vi "Control Panel.vi"(8 "error in (no error)":errorcluster, 11 "LCD Retarder in":refnum<class "LCD Retarder.lvclass">) -> (0 "error out":errorcluster, 3 "LCD Retarder out":refnum<class "LCD Retarder.lvclass">)   [LabVIEW 2017, in "LCD Retarder.lvclass"]
uses:
  LCD Retarder.lvclass
  LCD Retarder.lvclass/LCD Retarder.ctl
  <vilib>/DAQmx/write.llb/DAQmx Write (Analog DBL 1Chan 1Samp).vi
  <vilib>/DAQmx/create/channels.llb/DAQmx Create Channel (AO-Voltage-Basic).vi
  <vilib>/DAQmx/miscellaneous.llb/DAQmx Fill In Error Info.vi
  Main/Global/Flags.vi
  Utility Classes/Readable/Readable.lvclass
panel:
  in  "Analog \nOutput \nSync":bool
  in  "Alternate":bool
  in  "Frequency":dbl=0.01 min=0.01 max=6.0
  out "?":bool
  out "?":bool
  in  "Retardance 2":dbl
  in  "Retardance 1":dbl
  in  "stop":bool
  out "error":bool caption="Error"
  in  "Check for Instrument":bool
  out "Current Retardance":dbl[unit] caption="Retardance"
  out "Ready":bool
  in  "waveoptions":T1(radio) caption="Wave Options"
  in  "Wavelength":dbl[unit]=7.81e-07
  out "Title":string="LCD Retarder Control Program"
  in  "Zero":bool
  in  "Set\nRetardance":bool
  in  "Goto Retardance":dbl[unit]
  in  "Exit":bool
  # "and"
  # "at"
  # "Hz"
  # "between"
  # "Note from John: Analog Output #0 will toggle from 0 to 1 V in synch with this."
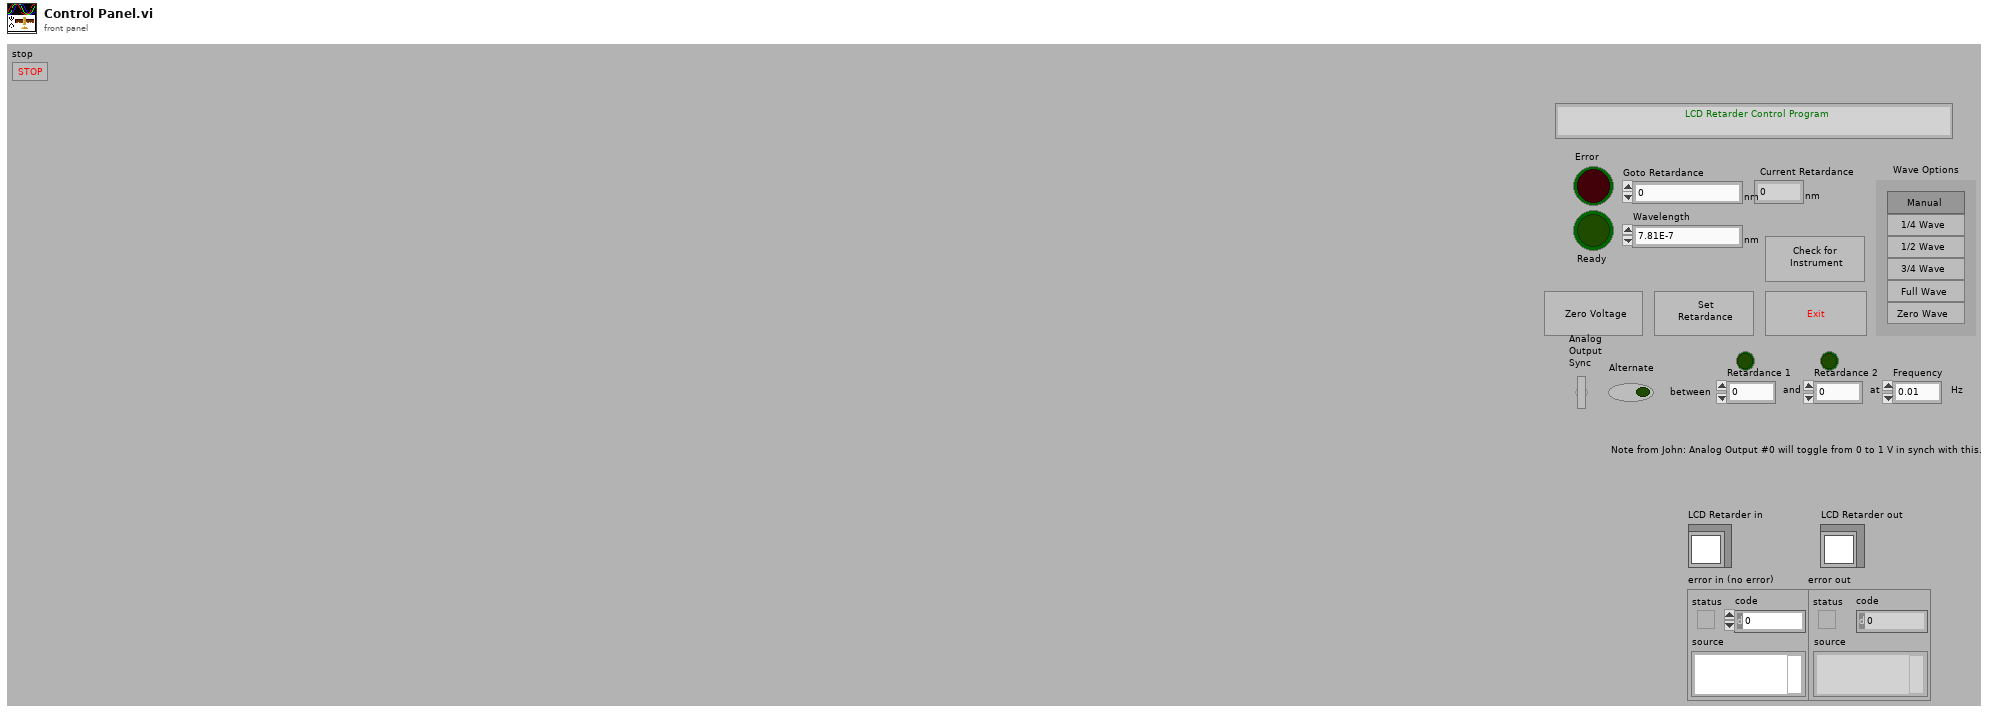
[diagram p1: front panel]
types:
  T1 = enum32{"Manual", "1/4 Wave", "1/2 Wave", "3/4 Wave", "Full Wave", "Zero Wave"}
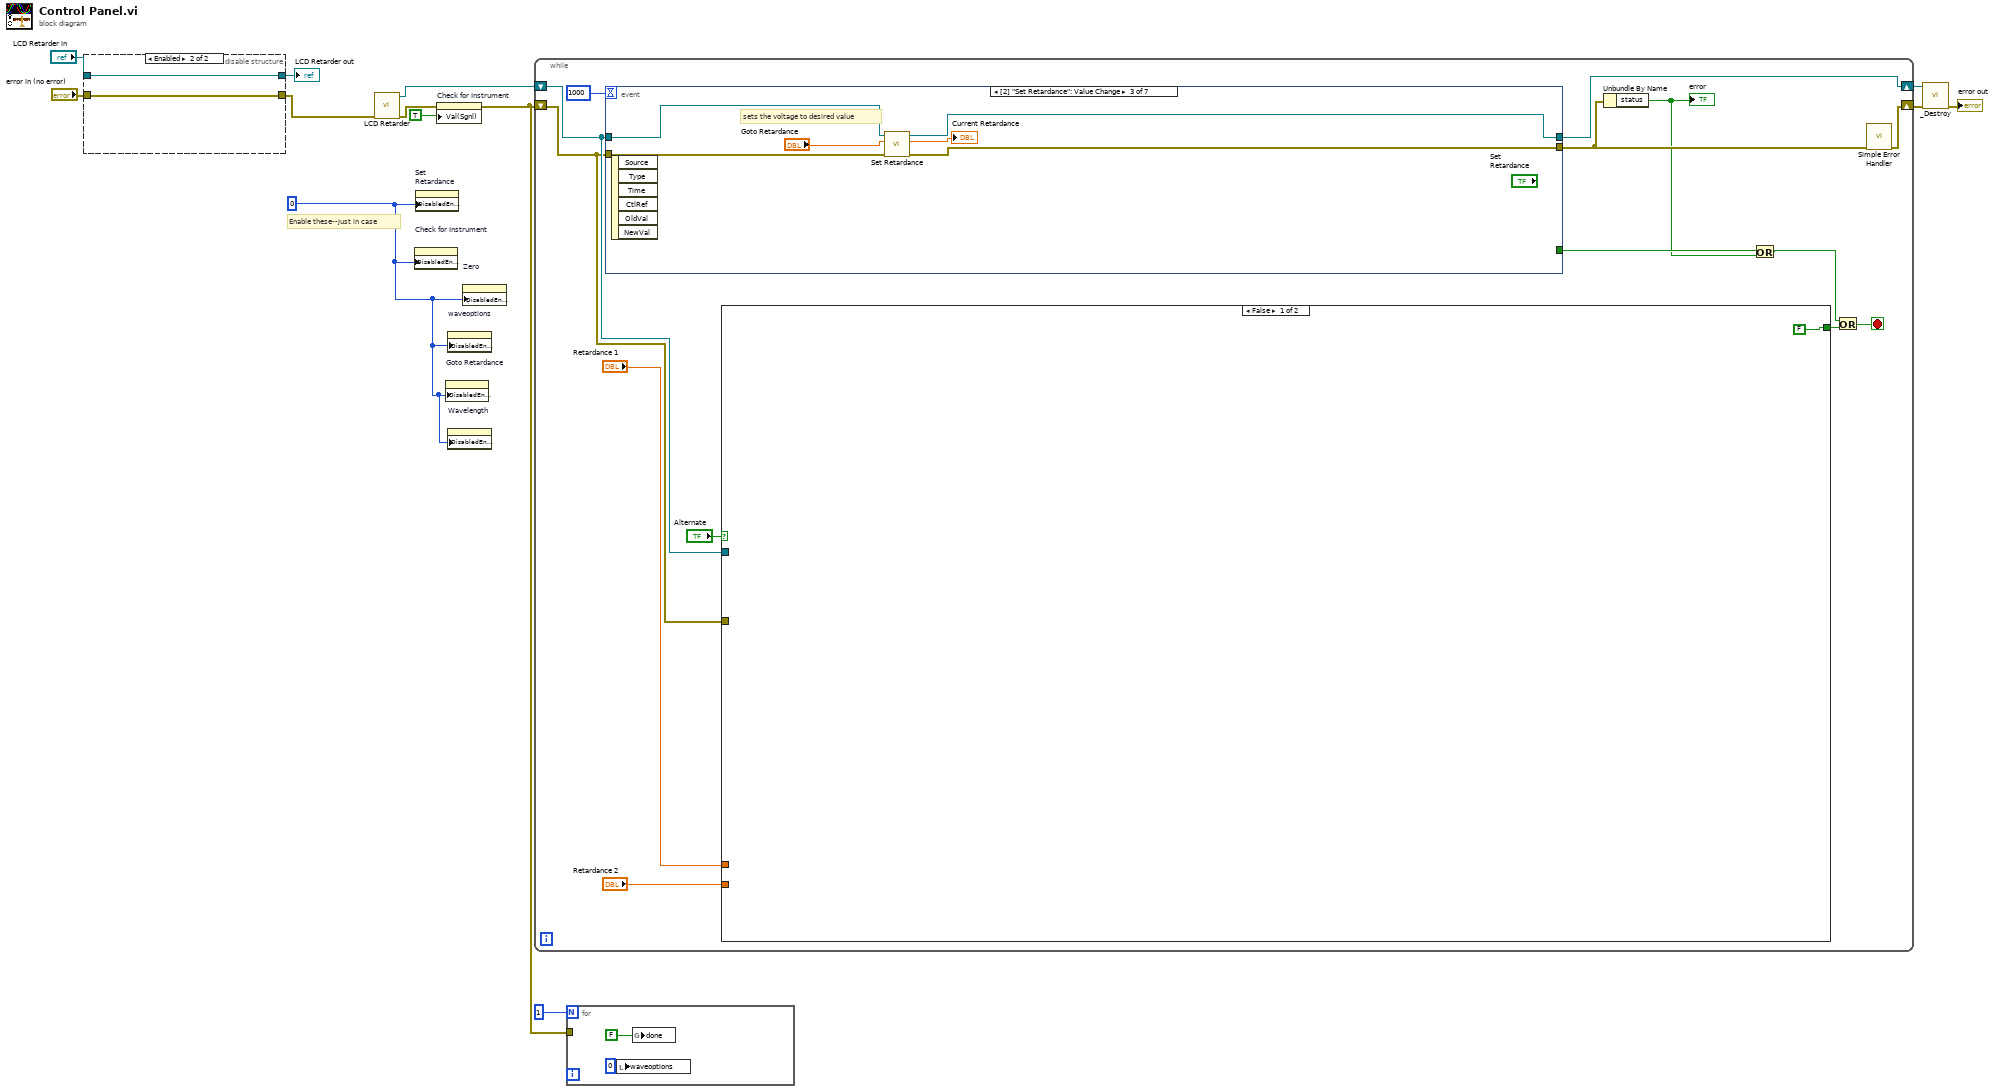
[diagram p0: block diagram]
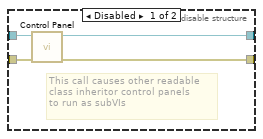
[diagram p2: hidden frame]
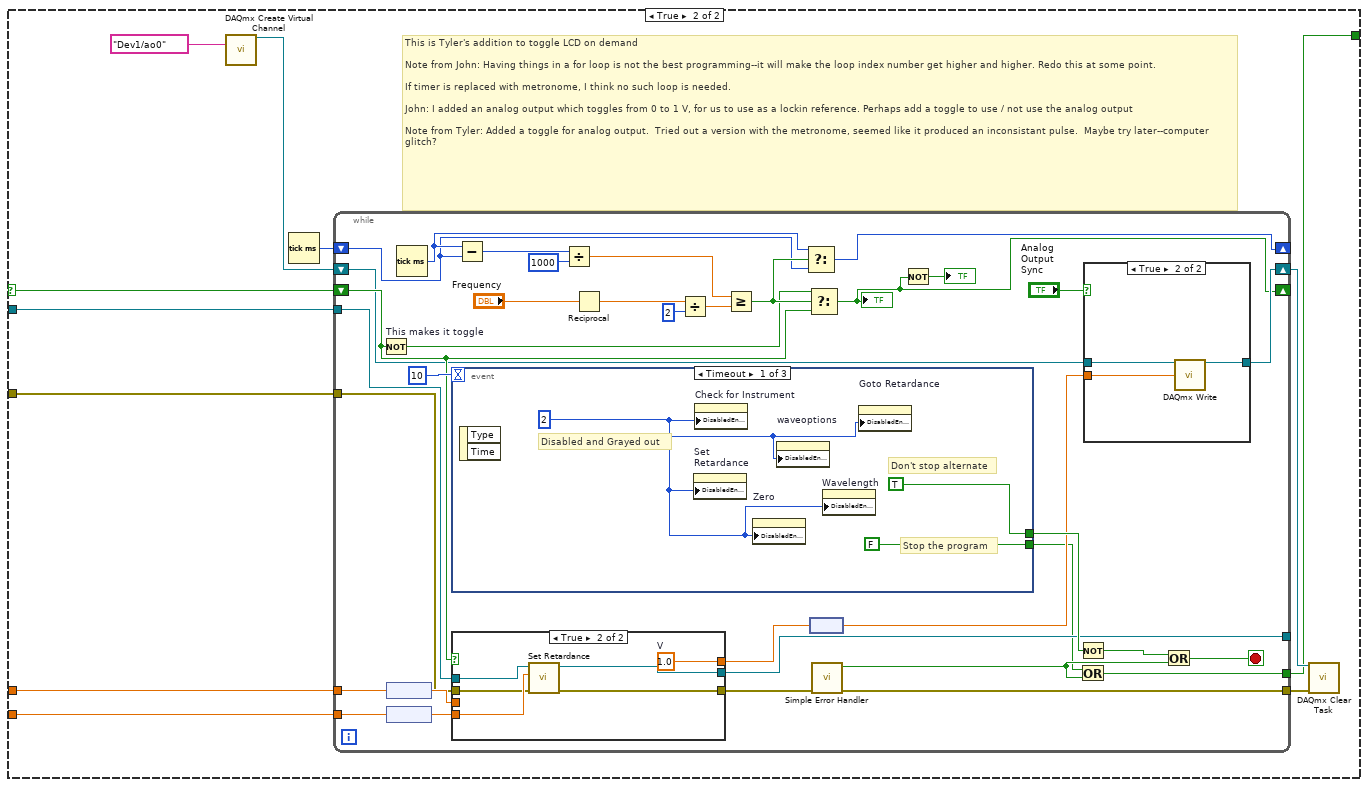
[diagram p3: hidden frame]
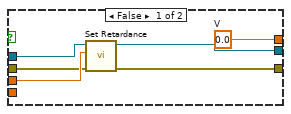
[diagram p5: hidden frame]
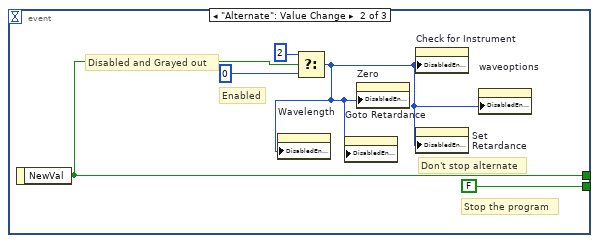
[diagram p6: hidden frame]
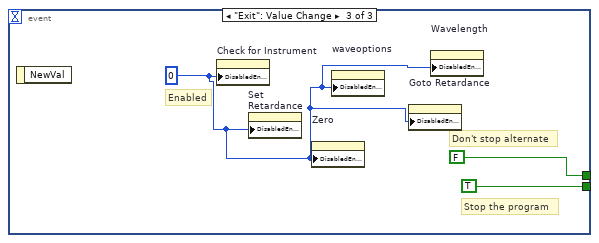
[diagram p7: hidden frame]
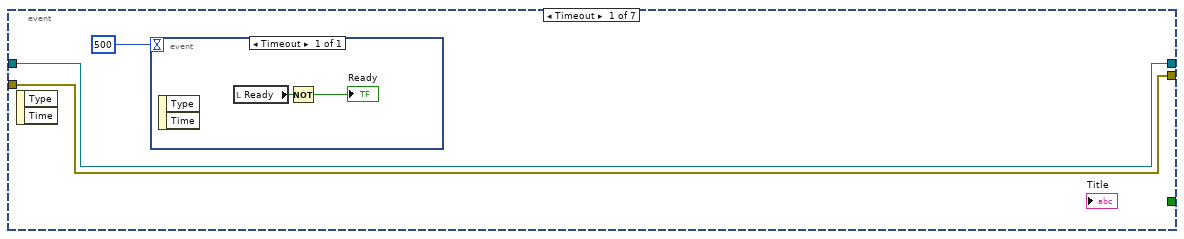
[diagram p8: hidden frame]
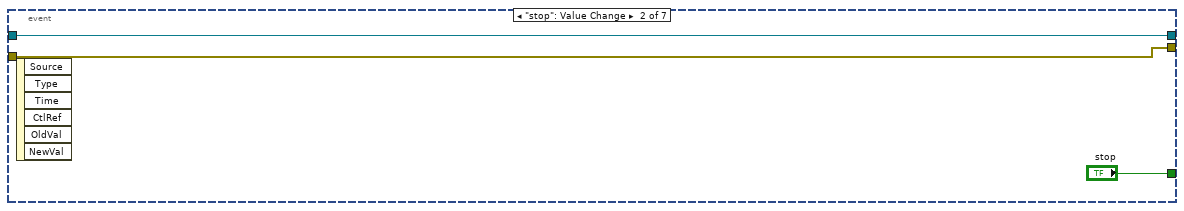
[diagram p9: hidden frame]
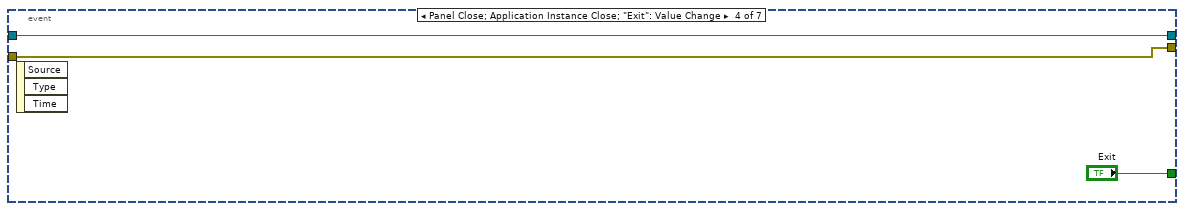
[diagram p10: hidden frame]
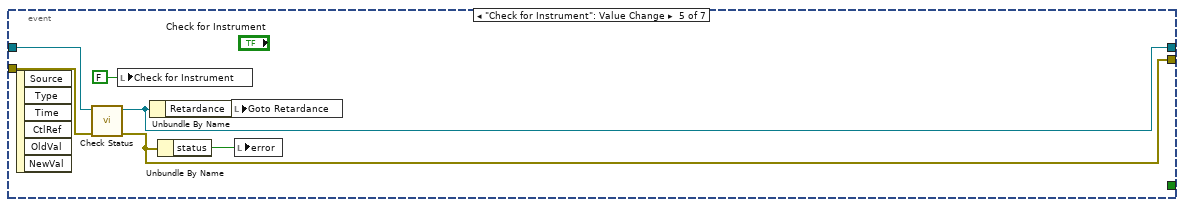
[diagram p11: hidden frame]
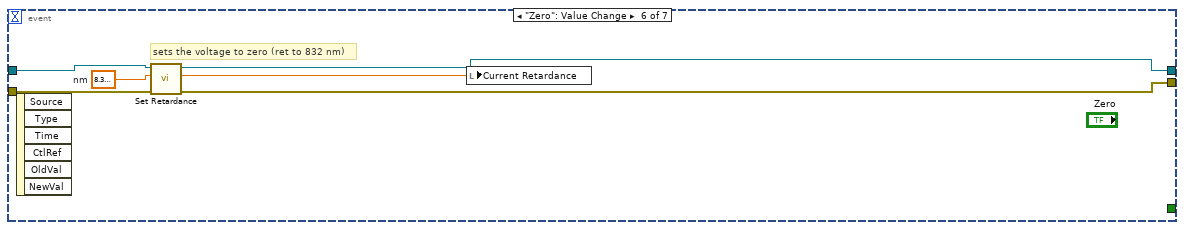
[diagram p12: hidden frame]
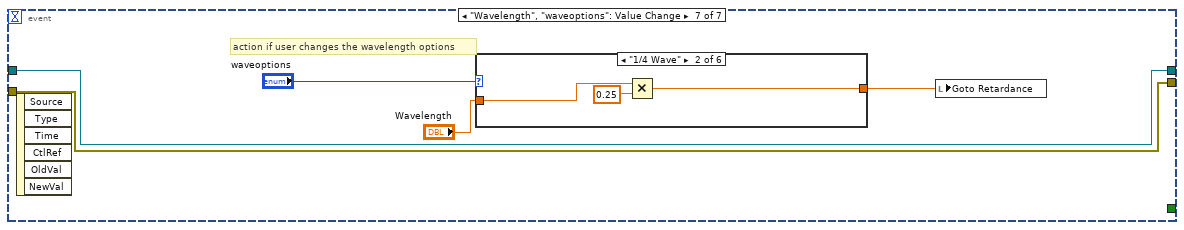
[diagram p13: hidden frame]
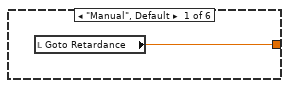
[diagram p14: hidden frame]
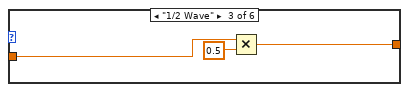
[diagram p15: hidden frame]
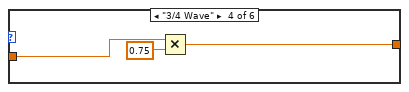
[diagram p16: hidden frame]
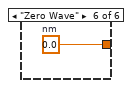
[diagram p18: hidden frame]
diagram:
  w1 = 0
  # "Enable these--just in case"
  n1 = disable-structure shown="Enabled" {
    disable-tunnel: [w17 w18] -> w13
    disable-tunnel: "error in (no error)" -> [w16 w18]
    disable-tunnel: "LCD Retarder in" -> [w15 w19]
    disable-tunnel: [w14 w19] -> w3
    frame Disabled {
      # "This call causes other readable\nclass inheritor control panels\nto run as subVIs"
      n2 = call-parent "Control Panel.vi"("error in (no error)"=w16, "Instrument in"=w15) -> ("error out"=w17:errorcluster, "Instrument out"=w14:refnum<class "LCD Retarder.lvclass">)  [unwired: 8 out]
    }
    frame Enabled {
    }
  }
  "LCD Retarder out" <- w3
  n3 = call "LCD Retarder.vi"("error in"=w13) -> ("errorOUT"=w5:errorcluster, "LCD out"=w2:refnum<class "LCD Retarder.lvclass">)  [unwired: 2 in, 7 out]
  n4 = property on="Check for Instrument" class="Bool (strict)"("DisabledEnum"=w1) -> ()  [unwired: 2 in, 2 out]
  n5 = property on="Set\nRetardance" class="Bool"("DisabledEnum"=w1) -> ()  [unwired: 2 in, 2 out]
  n6 = property on="Check for Instrument" class="Bool (strict)"(error in=w5, "Val(Sgnl)"=TRUE ("Value (Signaling)")) -> (error out=w4:errorcluster)  [unwired: 1 in, 1 out]
  n7 = property on="Goto Retardance" class="DigNum (strict)"("DisabledEnum"=w1) -> ()  [unwired: 2 in, 2 out]
  n8 = property on="waveoptions" class="RadioBtnsControl (strict)"("DisabledEnum"=w1) -> ()  [unwired: 2 in, 2 out]
  n9 = property on="Wavelength" class="DigNum (strict)"("DisabledEnum"=w1) -> ()  [unwired: 2 in, 2 out]
  n10 = property on="Zero" class="Bool"("DisabledEnum"=w1) -> ()  [unwired: 2 in, 2 out]
  n11 = while {
    shift-right: [w33] -> w12
    shift-left: w2 -> [w26]
    shift-right: [w31] -> w11
    shift-left: w4 -> [w25]
    stop <- w24 stop-if-true
    n12 = event shown="[2] \"Set Retardance\": Value Change" {
      selector: _ -> [_ _ _ _ _ _ _]
      dyn-events: _ -> [_ _ _ _ _ _ _]
      timeout: 1000 -> [_ _ _ _ _ _ _]
      tunnel: [_ "stop" _ "Exit" _ _ _] -> w21
      tunnel: [w110 w115 w121 w124 w127 w134 w141] -> w32
      tunnel: w25 -> [w110 w115 w119 w124 w132 w135 w141]
      tunnel: [w111 w114 w122 w125 w129 w133 w142] -> w33
      tunnel: w26 -> [w111 w114 w120 w125 w131 w136 w142]
      event Timeout {
        n13 = event-data() -> ()  [unwired: 3 out]
        n14 = event shown="[0] Timeout" {
          selector: _ -> [_]
          dyn-events: _ -> [_]
          timeout: 500 -> [_]
          event Timeout {
            n15 = event-data() -> ()  [unwired: 1 in, 2 out]
            n16 = local read "Ready"() -> (w113:bool)
            n17 = Not(x=w113) -> (.not. x?=→"Ready":bool)
          }
        }
      }
      event "stop": Value Change {
        n18 = event-data() -> ()  [unwired: 7 out]
      }
      event "Set\nRetardance": Value Change {
        # "sets the voltage to desired value"
        n19 = event-data() -> ()  [unwired: 7 out]
        n20 = call "Set Retardance.vi"("errorIN"=w119, "Retardance"="Goto Retardance", "LCD in"=w120) -> ("errorOUT"=w121:errorcluster, "Retardance out"=→"Current Retardance":dbl[unit], "LCD out"=w122:refnum<class "LCD Retarder.lvclass">)  [unwired: 6 out]
      }
      event Panel Close; Application Instance Close; "Exit": Value Change {
        n21 = event-data() -> ()  [unwired: 4 out]
      }
      event "Check for Instrument": Value Change {
        n22 = event-data() -> ()  [unwired: 7 out]
        n23 = call-dynamic "Check Status.vi"("error in (no error)"=w132, "LCD Retarder in"=w131) -> ("error out"=w127:errorcluster, "LCD Retarder out"=w129:refnum<class "LCD Retarder.lvclass">)  [unwired: 8 out]
        n24 = local write "Check for Instrument"(FALSE ("Check for Instrument")) -> ()
        n25 = Unbundle By Name(w129) -> ("Retardance"=w130:dbl[unit])
        n26 = Unbundle By Name(w127) -> ("status"=w126:bool)
        n27 = local write "Goto Retardance"(w130) -> ()
        n28 = local write "error"(w126) -> ()
      }
      event "Zero": Value Change {
        w137 = dbl[unit] 8.32e-07  # nm
        # "sets the voltage to zero (ret to 832 nm)"
        n29 = event-data() -> ()  [unwired: 7 out]
        n30 = call "Set Retardance.vi"("errorIN"=w135, "Retardance"=w137, "LCD in"=w136) -> ("errorOUT"=w134:errorcluster, "Retardance out"=w138:dbl[unit], "LCD out"=w133:refnum<class "LCD Retarder.lvclass">)  [unwired: 6 out]
        n31 = local write "Current Retardance"(w138) -> ()
      }
      event "Wavelength", "waveoptions": Value Change {
        # "action if user changes the wavelength options"
        n32 = event-data() -> ()  [unwired: 7 out]
        n33 = case shown="\"1/4 Wave\"" "waveoptions" {
          tunnel: "Wavelength" -> [_ w147 w150 w153 w154 _]
          tunnel: [w144 w145 w148 w151 w154 w155] -> w143
          frame "Manual", Default {
            n34 = local read "Goto Retardance"() -> (w144:dbl[unit])
          }
          frame "1/4 Wave" {
            n35 = Multiply(x=w147, y=0.25) -> (x*y=w145:dbl[unit])
          }
          frame "1/2 Wave" {
            n36 = Multiply(x=w150, y=0.5) -> (x*y=w148:dbl[unit])
          }
          frame "3/4 Wave" {
            n37 = Multiply(x=w153, y=0.75) -> (x*y=w151:dbl[unit])
          }
          frame "Full Wave" {
          }
          frame "Zero Wave" {
            w155 = dbl[unit] 0.0  # nm
          }
        }
        n38 = local write "Goto Retardance"(w143) -> ()
      }
    }
    n39 = case shown="False" "Alternate" {
      selector: "Alternate" -> [_ w44]
      tunnel: "Retardance 1" -> [_ w43]
      tunnel: "Retardance 2" -> [_ w42]
      tunnel: w26 -> [_ w37]
      tunnel: w25 -> [_ w36]
      tunnel: [FALSE w35] -> w23
      frame False {
      }
      frame True {
        # "This is Tyler's addition to toggle LCD on demand\n\nNote from John: Having things in a for loop is not the best programming--it will make the loop index number get higher and higher. Redo this at some point.\n\nIf timer is replaced with metronome, I think no such loop is needed.\n\nJohn: I added an analog output which toggles from 0 to 1 V, for us to use as a lockin reference. Perhaps add a toggle to use / not use the analog output\n\nNote from Tyler: Added a toggle for analog output.  Tried out a version with the metronome, seemed like it produced an inconsistant pulse.  Maybe try later--computer glitch?"
        n40 = call-poly <vilib>:"DAQmx Create Virtual Channel.vi"("physical channels"=tag "Dev1/ao0") -> ("task out"=w40:refnum<k21>)  [unwired: 13 in, 1 out]
        n41 = Tick Count (ms)() -> (millisecond timer value=w45:u32)
        n42 = while {
          shift-right: [w69] -> _
          shift-left: w45 -> [w70]
          shift-right: [w57] -> _
          shift-left: w44 -> [w68]
          tunnel: [w67] -> _
          tunnel: [w51] -> w38
          tunnel: w43 -> [w66]
          tunnel: w42 -> [w65]
          tunnel: w37 -> [w63]
          tunnel: w36 -> [w64]
          shift-right: [w60] -> w39
          shift-left: w40 -> [w59]
          tunnel: [w48] -> w35
          stop <- w49 stop-if-true
          n43 = Not "This makes it toggle"(x=w68) -> (.not. x?=w72:bool)
          n44 = node(w66) -> (w79:dbl[unit])
          n45 = node(w65) -> (w78:dbl[unit])
          n46 = Tick Count (ms)() -> (millisecond timer value=w74:u32)
          n47 = event shown="[0] Timeout" {
            selector: _ -> [_ _ _]
            dyn-events: _ -> [_ _ _]
            timeout: 10 -> [_ _ _]
            tunnel: [TRUE w103 FALSE] -> w80
            tunnel: [FALSE FALSE TRUE] -> w46
            event Timeout {
              w98 = 2
              # "Don't stop alternate"
              # "Stop the program"
              # "Disabled and Grayed out"
              n48 = event-data() -> ()  [unwired: 1 in, 2 out]
              n49 = property on="Set\nRetardance" class="Bool"("DisabledEnum"=w98) -> ()  [unwired: 2 in, 2 out]
              n50 = property on="Check for Instrument" class="Bool (strict)"("DisabledEnum"=w98) -> ()  [unwired: 2 in, 2 out]
              n51 = property on="Zero" class="Bool"("DisabledEnum"=w98) -> ()  [unwired: 2 in, 2 out]
              n52 = property on="waveoptions" class="RadioBtnsControl (strict)"("DisabledEnum"=w98) -> ()  [unwired: 2 in, 2 out]
              n53 = property on="Wavelength" class="DigNum (strict)"("DisabledEnum"=w98) -> ()  [unwired: 2 in, 2 out]
              n54 = property on="Goto Retardance" class="DigNum (strict)"("DisabledEnum"=w98) -> ()  [unwired: 2 in, 2 out]
            }
            event "Alternate": Value Change {
              # "Enabled"
              # "Disabled and Grayed out"
              # "Don't stop alternate"
              # "Stop the program"
              n55 = event-data() -> ("NewVal"=w103:bool)  [unwired: 1 in]
              n56 = Select(t=2, s=w103, f=0) -> (s? t:f=w101:i32)
              n57 = property on="Wavelength" class="DigNum (strict)"("DisabledEnum"=w101) -> ()  [unwired: 2 in, 2 out]
              n58 = property on="Goto Retardance" class="DigNum (strict)"("DisabledEnum"=w101) -> ()  [unwired: 2 in, 2 out]
              n59 = property on="Zero" class="Bool"("DisabledEnum"=w101) -> ()  [unwired: 2 in, 2 out]
              n60 = property on="Check for Instrument" class="Bool (strict)"("DisabledEnum"=w101) -> ()  [unwired: 2 in, 2 out]
              n61 = property on="Set\nRetardance" class="Bool"("DisabledEnum"=w101) -> ()  [unwired: 2 in, 2 out]
              n62 = property on="waveoptions" class="RadioBtnsControl (strict)"("DisabledEnum"=w101) -> ()  [unwired: 2 in, 2 out]
            }
            event "Exit": Value Change {
              w106 = 0
              # "Enabled"
              # "Don't stop alternate"
              # "Stop the program"
              n63 = event-data() -> ()  [unwired: 1 in, 1 out]
              n64 = property on="Check for Instrument" class="Bool (strict)"("DisabledEnum"=w106) -> ()  [unwired: 2 in, 2 out]
              n65 = property on="Set\nRetardance" class="Bool"("DisabledEnum"=w106) -> ()  [unwired: 2 in, 2 out]
              n66 = property on="Zero" class="Bool"("DisabledEnum"=w106) -> ()  [unwired: 2 in, 2 out]
              n67 = property on="waveoptions" class="RadioBtnsControl (strict)"("DisabledEnum"=w106) -> ()  [unwired: 2 in, 2 out]
              n68 = property on="Goto Retardance" class="DigNum (strict)"("DisabledEnum"=w106) -> ()  [unwired: 2 in, 2 out]
              n69 = property on="Wavelength" class="DigNum (strict)"("DisabledEnum"=w106) -> ()  [unwired: 2 in, 2 out]
            }
          }
          n70 = case shown="True" w68 {
            tunnel: w79 -> [w90 _]
            tunnel: [w91 w97] -> w67
            tunnel: [w89 w96] -> w52
            tunnel: w78 -> [_ w95]
            tunnel: w64 -> [w87 w93]
            tunnel: w63 -> [w88 w94]
            tunnel: [w86 w92] -> w61
            frame False {
              w86 = dbl[unit] 0.0  # V
              n71 = call "Set Retardance.vi"("errorIN"=w87, "Retardance"=w90, "LCD in"=w88) -> ("errorOUT"=w89:errorcluster, "LCD out"=w91:refnum<class "LCD Retarder.lvclass">)  [unwired: 6 in, 1 out]
            }
            frame True {
              w92 = dbl[unit] 1.0  # V
              n72 = call "Set Retardance.vi"("errorIN"=w93, "Retardance"=w95, "LCD in"=w94) -> ("errorOUT"=w96:errorcluster, "LCD out"=w97:refnum<class "LCD Retarder.lvclass">)  [unwired: 6 in, 1 out]
            }
          }
          n73 = Subtract(x=w74, y=w70) -> (x-y=w77:u32)
          n74 = Divide(x=w77, y=1000) -> (x/y=w75:dbl)
          n75 = Reciprocal(x="Frequency") -> (1/x=w55:dbl)
          n76 = Divide(x=w55, y=2) -> (x/y=w56:dbl)
          n77 = Greater Or Equal?(x=w75, y=w56) -> (x >= y?=w73:bool)
          n78 = Select(t=w74, s=w73, f=w70) -> (s? t:f=w69:u32)
          n79 = Select(t=w72, s=w73, f=w68) -> (s? t:f=w57:bool)
          "?" <- w57
          n80 = node(w61) -> (w62:dbl)
          n81 = call <vilib>:"Simple Error Handler.vi"("error in (no error)"=w52) -> ("error?"=w47:bool, "error out"=w51:errorcluster)  [unwired: 1 in, 6 out]
          n82 = Not(x=w57) -> (.not. x?=→"?":bool)
          n83 = Not(x=w80) -> (.not. x?=w50:bool)
          n84 = Or(x=w46, y=w47) -> (x .or. y?=w48:bool)
          n85 = case shown="True" "Analog \nOutput \nSync" {
            tunnel: w62 -> [_ w85]
            tunnel: [w82 w84] -> w60
            tunnel: w59 -> [w82 w83]
            frame False {
            }
            frame True {
              n86 = call-poly <vilib>:"DAQmx Write.vi"("task/channels in"=w83, "data"=w85) -> ("task out"=w84:refnum<k21>)  [unwired: 11 in, 2 out]
            }
          }
          n87 = Or(x=w50, y=w47) -> (x .or. y?=w49:bool)
        }
        n88 = call <vilib>:"DAQmx Clear Task.vi"("task in"=w39, "error in"=w38) -> ()  [unwired: 13 in, 1 out]
      }
    }
    n89 = Unbundle By Name(w32) -> ("status"=w20:bool)
    "error" <- w20
    n90 = Or(x=w21, y=w20) -> (x .or. y?=w22:bool)
    n91 = Or(x=w22, y=w23) -> (x .or. y?=w24:bool)
    n92 = call <vilib>:"Simple Error Handler.vi"("error in (no error)"=w32) -> ("error out"=w31:errorcluster)  [unwired: 1 in, 7 out]
  }
  n93 = for {
    N: 1 -> [_]
    tunnel: w4 -> [_]
    n94 = local write "waveoptions"(0) -> ()
    n95 = global write "Flags.vi" "done"(FALSE) -> ()
  }
  n96 = call-dynamic "_Destroy.vi"("error in (no error)"=w11, "LCD Retarder in"=w12) -> ("error out"=→"error out":errorcluster)  [unwired: 9 out]
